vi "intersectionVectors.vi"(10 "vector2":dbl[](array[numeric]), 11 "vector1":dbl[](array[numeric])) -> (1 "elements":dbl[](array[numeric]), 3 "vector1 indices":i32[](array[numeric]))   [LabVIEW 2017]
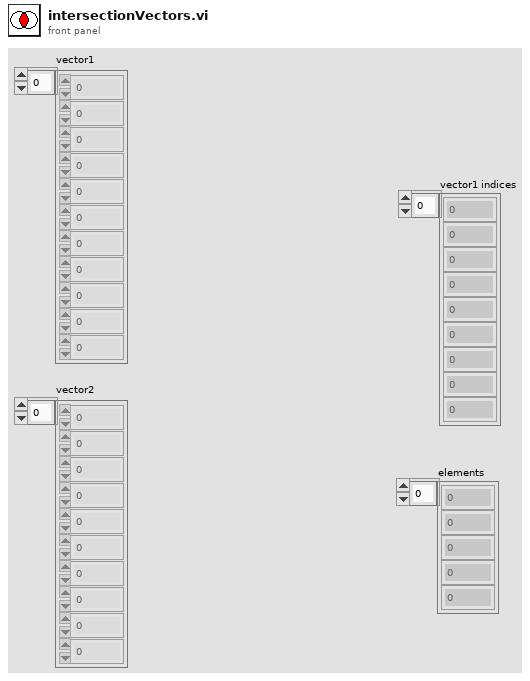
[diagram p1: front panel]
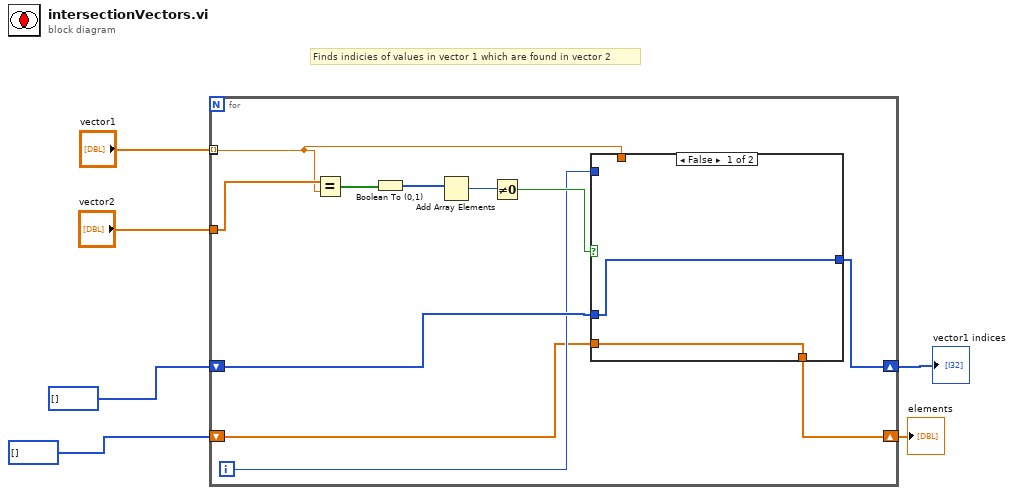
[diagram p0: block diagram]
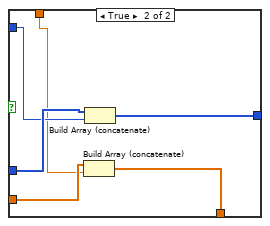
[diagram p2: hidden frame]
diagram:
  # "Finds indicies of values in vector 1 which are found in vector 2"
  n1 = for {
    tunnel: [w8] -> _ mode=indexing
    tunnel: "vector1" -> [w8] mode=indexing
    tunnel: "vector2" -> [w17]
    shift-right: [w11] -> w3
    shift-left: i32[] [] ("initialized\narray") -> [w12]
    shift-right: [w7] -> w1
    shift-left: i32[] [] ("initialized\narray 2") -> [w9]
    i -> [w10]
    n2 = Equal?(x=w17, y=w8) -> (x = y?=w16:bool[])
    n3 = Boolean To (0,1)(Boolean=w16) -> (0, 1=w15:i16[])
    n4 = Add Array Elements(numeric array=w15) -> (sum=w14:i16)
    n5 = Not Equal To 0?(x=w14) -> (x != 0?=w13:bool)
    n6 = case shown="False" w13 {
      tunnel: w12 -> [w19 w25]
      tunnel: [w19 w24] -> w11
      tunnel: w10 -> [_ w23]
      tunnel: w9 -> [w18 w22]
      tunnel: w8 -> [_ w21]
      tunnel: [w18 w20] -> w7
      frame False {
      }
      frame True {
        n7 = Build Array (concatenate)(w22, w21) -> (w20:dbl[])
        n8 = Build Array (concatenate)(w25, w23) -> (w24:i32[])
      }
    }
  }
  "vector1 indices" <- w3
  "elements" <- w1
